vi "LVPortUnBindProperties.vi"(9 "Controls To Bind":refnum<vi>[](array[refnum]), 10 "Control To Bind":refnum<vi>, 11 "pID":string) -> ()   [LabVIEW 2017]
uses:
  LVPortControlBindingInfoType.ctl
  LVPortControlBindingDirectionEnum.ctl
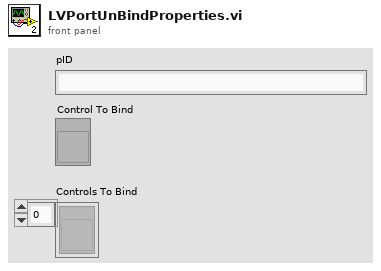
[diagram p1: front panel]
types:
  T1 = typedef "Dictionary Object RefNum__ogtk.ctl" = refnum<k1>
  T2 = typedef "LVPortControlBindingInfoType.ctl" = cluster{"Bound Control":refnum<vi>, "Name":string, "Direction":T3}
  T3 = typedef "LVPortControlBindingDirectionEnum.ctl" = enum16{"BiDirectional", "ToMatlab", "ToLabview"}
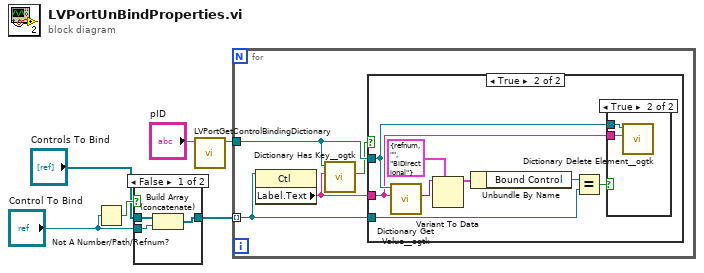
[diagram p0: block diagram]
diagram:
  n1 = Not A Number/Path/Refnum?(number/path/refnum="Control To Bind") -> (NaN/Path/Refnum?=w6:bool)
  n2 = case shown="False" w6 {
    tunnel: "Controls To Bind" -> [w9 w10]
    tunnel: "Control To Bind" -> [w8 _]
    tunnel: [w7 w10] -> w2
    frame False {
      n3 = Build Array (concatenate)(w9, w8) -> (w7:refnum<vi>[])
    }
    frame True {
    }
  }
  n4 = call "LVPortGetControlBindingDictionary.vi"("pID"="pID") -> ("Refnum out"=w1:T1)  [unwired: 10 in]
  n5 = for {
    tunnel: w2 -> [w14] mode=indexing
    tunnel: w1 -> [w12]
    n6 = property class="Ctl"(reference=w14) -> ("Label.Text"=w13:string)  [unwired: 1 in, 2 out]
    n7 = call <userlib>:"Dictionary Has Key__ogtk.vi"("key"=w13, "dictionary"=w12) -> ("Has Key?"=w11:bool)  [unwired: 7 in, 2 out]
    n8 = case shown="True" w11 {
      tunnel: w14 -> [_ w16]
      tunnel: w13 -> [_ w20]
      tunnel: w12 -> [_ w21]
      frame False {
      }
      frame True {
        n9 = call <userlib>:"Dictionary Get Value__ogtk.vi"("key"=w20, "dictionary"=w21) -> ("value"=w22:variant)  [unwired: 6 in, 3 out]
        n10 = Variant To Data(type=T2 {"Bound Control"=refnum, "Name"="", "Direction"=enum."BiDirectional"} ("Control Binding Info"), Variant=w22) -> (data=w18:T2)  [unwired: 1 in, 1 out]
        n11 = Unbundle By Name(w18) -> ("Bound Control"=w17:refnum<vi>)
        n12 = Equal?(x=w17, y=w16) -> (x = y?=w15:bool)
        n13 = case shown="True" w15 {
          tunnel: w20 -> [_ w24]
          tunnel: w21 -> [_ w23]
          frame False {
          }
          frame True {
            n14 = call <userlib>:"Dictionary Delete Element__ogtk.vi"("key"=w24, "dictionary"=w23) -> ()  [unwired: 8 in, 2 out]
          }
        }
      }
    }
  }
